vi "Format Codes.vi"(11 "List type":T1 caption="HLP_Format Code List Type") -> (2 "Caption":string, 3 "Item Names":string[][](array[string]))   [LabVIEW 2018, in "Numeric Data Type.lvclass"]
uses:
  Numeric Data Type.lvclass
  Format Code Type List Enum.ctl
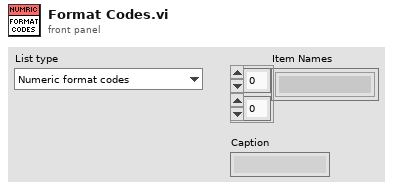
[diagram p1: front panel]
types:
  T1 = typedef "Numeric Data Type.lvclass/Format Code Type List Enum.ctl" = enum16{"Numeric format codes", "Relative time format codes", "Absolute time format codes"}
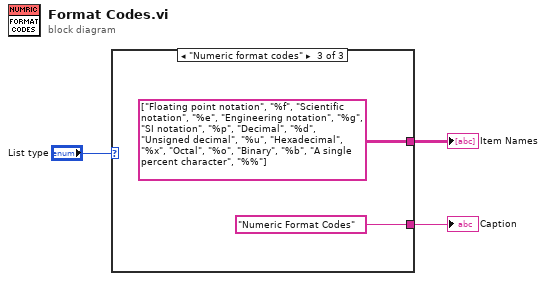
[diagram p0: block diagram]
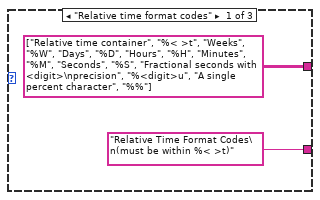
[diagram p2: hidden frame]
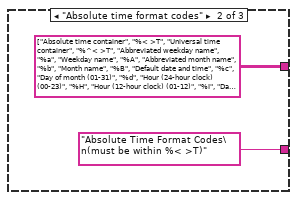
[diagram p3: hidden frame]
diagram:
  n1 = case shown="\"Numeric format codes\"" "List type" {
    tunnel: [string[][] [["Relative time container", "%< >t"], ["Weeks", "%W"], ["Days", "%D"], ["Hours", "%H"], ["Minutes", "%M"], ["Seconds", "%S"], ["Fractional seconds with <digit>\nprecision", "%<digit>u"], ["A single percent character", "%%"]] ("Item Names 2") string[][] [["Absolute time container", "%< >T"], ["Universal time container", "%^< >T"], ["Abbreviated weekday name", "%a"], ["Weekday name", "%A"], ["Abbreviated month name", "%b"], ["Month name", "%B"], ["Default date and time", "%c"], ["Day of month (01-31)", "%d"], ["Hour (24-hour clock) (00-23)", "%H"], ["Hour (12-hour clock) (01-12)", "%I"], ["Day of year (001-366)", "%j"], ["Month number (01-12)", "%m"], ["Minute (00-59)", "%M"], ["AM or PM flag", "%p"], ["Seconds (00-59)", "%S"], ["Fractional seconds with <digit>\nprecision", "%<digit> u"], ["Week number (00-53) with\nSunday as the first day of week 1", "%U"], ["Weekday number (0-6)", "%w"], ["Week number (00-53) with\nMonday as the first day of week 1", "%W"], ["Locale date", "%x"], ["Locale time", "%X"], ["Year within century (00-99)", "%y"], ["Year including century", "%Y"], ["Time zone", "%Z"]] ("Item Names 3") string[][] [["Floating point notation", "%f"], ["Scientific notation", "%e"], ["Engineering notation", "%g"], ["SI notation", "%p"], ["Decimal", "%d"], ["Unsigned decimal", "%u"], ["Hexadecimal", "%x"], ["Octal", "%o"], ["Binary", "%b"], ["A single percent character", "%%"]] ("Item Names")] -> w2
    tunnel: ["Relative Time Format Codes\n(must be within %< >t)" ("Caption.Text") "Absolute Time Format Codes\n(must be within %< >T)" ("Caption.Text") "Numeric Format Codes" ("Caption.Text")] -> w3
    frame "Relative time format codes" {
    }
    frame "Absolute time format codes" {
    }
    frame "Numeric format codes" {
    }
  }
  "Caption" <- w3
  "Item Names" <- w2
